vi "Get Size.vi"(8 "error in (no error)":errorcluster, 11 "Transfer Configuration in":refnum<class "Configuration.Transfer.lvclass">) -> (0 "error out":errorcluster, 2 "size in bytes":u64, 3 "Transfer Configuration out":refnum<class "Configuration.Transfer.lvclass">)   [LabVIEW 2016, in "Configuration.Transfer.lvclass"]
uses:
  Configuration.Transfer.lvclass
  Configuration.Transfer.lvclass/Configuration.Transfer.ctl
  Configuration.Channel/Configuration.Channel.lvclass
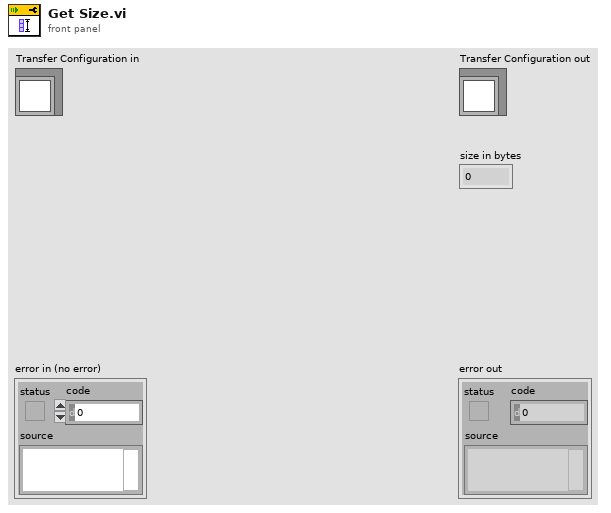
[diagram p1: front panel]
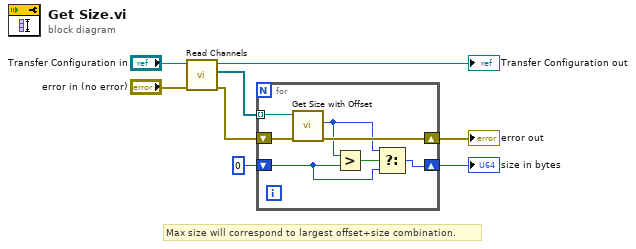
[diagram p0: block diagram]
diagram:
  # "Max size will correspond to largest offset+size combination."
  n1 = call "Read Channels.vi"("error in (no error)"="error in (no error)", "Configuration.Transfer in"="Transfer Configuration in") -> ("error out"=w7:errorcluster, "Channels"=w8:refnum<class "Configuration.Channel.lvclass">[], "Configuration.Transfer out"=→"Transfer Configuration out":refnum<class "Configuration.Transfer.lvclass">)  [unwired: 7 in]
  n2 = for {
    tunnel: w8 -> [w14] mode=indexing
    shift-right: [w10] -> w2
    shift-left: w7 -> [w15]
    shift-right: [w11] -> w1
    shift-left: u64 0 -> [w12]
    n3 = call "Get Size with Offset.vi"("error in (no error)"=w15, "Channel Configuration in"=w14) -> ("error out"=w10:errorcluster, "size+offset in bytes"=w9:u64)  [unwired: 7 in, 1 out]
    n4 = Greater?(x=w9, y=w12) -> (0:w13:bool)
    n5 = Select(t=w9, s=w13, f=w12) -> (s? t:f=w11:u64)
  }
  "error out" <- w2
  "size in bytes" <- w1
